vi "BSCAN_DEMO00_init_xc7z020_clg400.vi"() -> ()   [LabVIEW 2017]
doc: "Copyright © 2024 SalDigi Oy, all rights reserved."
uses:
  Saldigi_protocol_library.lvlibp/HAL/HAL_version_typedef.ctl
  Saldigi_protocol_library.lvlibp/BSCAN_bitstream/private/BSCAN_INSTRUCTION_OPCODE_typedef.ctl
  Saldigi_protocol_library.lvlibp/BSCAN_bitstream/BSCAN_typedef.ctl
  Saldigi_protocol_library.lvlibp/BSCAN_bitstream/BSCAN_state_typedef.ctl
  Saldigi_protocol_library.lvlibp/BSCAN_bitstream/simultaneous/BSCAN_extest_dataToInject.ctl
  Saldigi_protocol_library.lvlibp
panel:
  in  "TAPs OPCODE array (use only BYPASS or EXTEST here)":T1[](array[typedef])=[enum."BYPASS", enum."EXTEST"]
  in  "HAL Version":T2=enum."FTn232H"
  in  "Init output rate":dbl=1000000.0 format="%^#_6g"
  in  "Start V2 Server":bool
  out "shift-IR OK":bool
  out "ID registers from BSDL out (string)":string[](array[string])
  out "ID registers out (U32)":u32[](array[numeric]) format="%032b"
  in  "CHAINn name in":string(combo)="chain0"
  in  "Parameter string":string(combo)="FTERYEPB"
  in  "TDO-in channel name":string(combo)="D3"
  in  "TCK channel name":string(combo)="D0"
  in  "TDI channel name":string(combo)="D1"
  in  "TMS channel name":string(combo)="D6"
  in  "output rate":dbl=10000000.0 format="%^#_6g"
  in  "BSDL files in":path[](array[path])=[path "C:/bitstream/zynq7000_arm_dap.bsd", path "C:/bitstream/xc7z020_clg400.bsd"]
  out "error out":errorcluster
  in  "error in":errorcluster
  out "ALL TAPs IDCODE OK":bool
  # "First TAP in CHAINn is on array index[0]."
  # "The combo boxes below include examples for DAQmx and FTn232H. Edit these to suit your\nsystem."
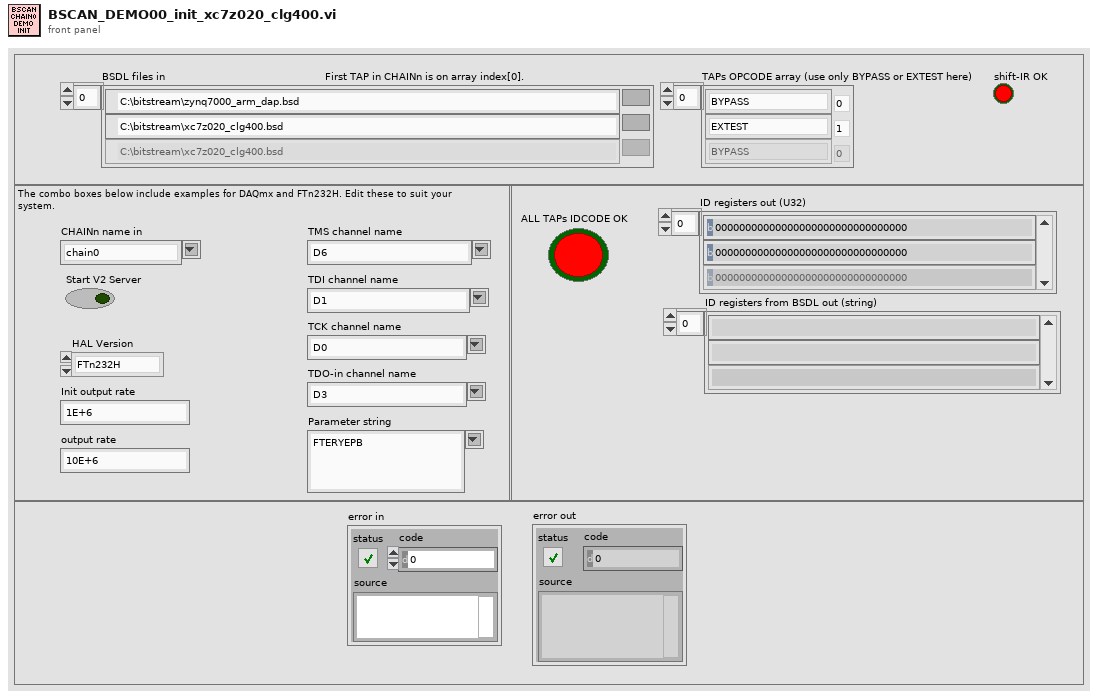
[diagram p1: front panel]
types:
  T1 = typedef "Saldigi_protocol_library.lvlibp/BSCAN_INSTRUCTION_OPCODE_typedef.ctl" = enum16{"BYPASS", "EXTEST", "PRELOAD", "SAMPLE", "CLAMP", "HIGHZ", "INTEST", "RUNBIST", "USERCODE", "IDCODE"}
  T2 = typedef "Saldigi_protocol_library.lvlibp/HAL_version_typedef.ctl" = enum16{"DAQmx V1", "DAQmx V2", "FTn232H", "BSCAN V1", "DAQmx V1.1", "DAQmx V2.1", "J-LINK BSCAN", "BSCAN V2"}
  T3 = typedef "Saldigi_protocol_library.lvlibp/BSCAN_typedef.ctl" = cluster{"TMS":bool[], "TDI":bool[], "TCK":bool[], "TDO-in":bool[], "clocked bits":i32, "output rate":dbl, "TMS channel name":string, "TDI channel name":string, "TCK channel name":string, "TDO-in channel name":string, "Parameter string":string, "String array":string[], "State":T4, "CHAINn":string, "Version":T2, "V2 Server queue":refnum<queue>, "V2 max client \ndata array length":i32}
  T4 = typedef "Saldigi_protocol_library.lvlibp/BSCAN_state_typedef.ctl" = enum16{"Test-Logic-Reset", "Run-Test/Idle", "Select DR-Scan", "Capture-DR", "Shift-DR", "Exit1-DR", "Pause-DR", "Exit2-DR", "Update-DR", "Select-IR-Scan", "Capture-IR", "Shift-IR", "Exit1-IR", "Pause-IR", "Exit2-IR", "Update-IR"}
  T5 = cluster{"CHAINn/TARGETn/PORTn in":string[], "port states in":bool[], "port driver states in":enum16{"Enable driver", "Disable driver", "Read"}[]}
  T6 = enum16{"Enable driver", "Disable driver", "Read"}[]
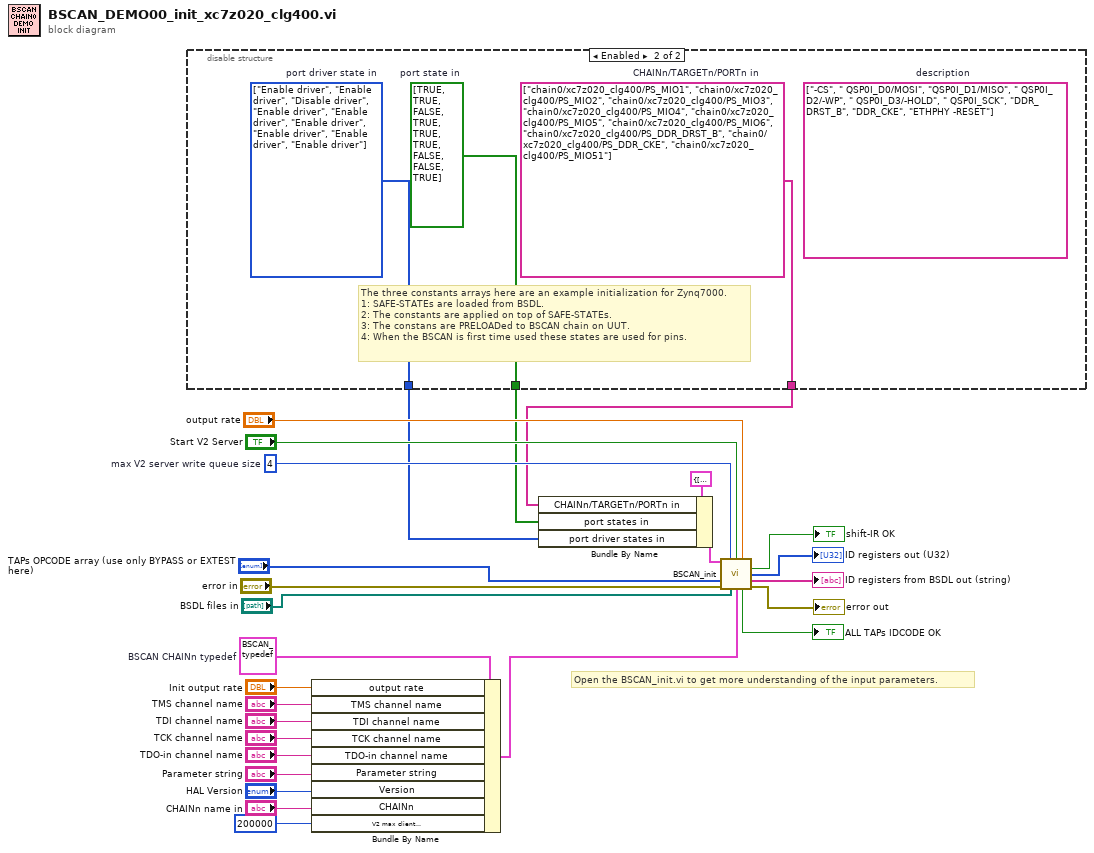
[diagram p0: block diagram]
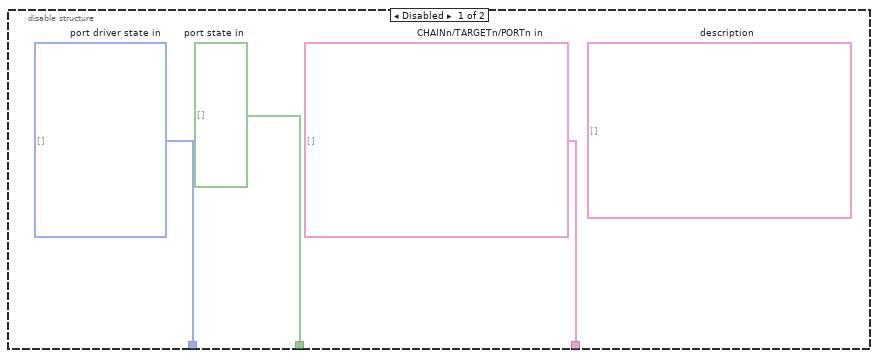
[diagram p2: hidden frame]
diagram:
  w2 = T3 {"TMS"=[], "TDI"=[], "TCK"=[], "TDO-in"=[], "clocked bits"=0, "output rate"=0.0, "TMS channel name"="", "TDI channel name"="", "TCK channel name"="", "TDO-in channel name"="", "Parameter string"="", "String array"=[], "State"=enum."Test-Logic-Reset", "CHAINn"="chain0", "Version"=enum."FTn232H", "V2 Server queue"=refnum, "V2 max client \ndata array length"=0}  # BSCAN CHAINn typedef
  w21 = 4  # max V2 server write queue size
  # "Open the BSCAN_init.vi to get more understanding of the input parameters."
  n1 = disable-structure shown="Enabled" {
    disable-tunnel: [w30 w33] -> w9
    disable-tunnel: [w29 w32] -> w8
    disable-tunnel: [w28 w31] -> w7
    frame Disabled {
      (unwired) string[] []  # description
      w29 = bool[] []  # port state in
      w28 = T6 [] items=["Enable driver", "Disable driver", "Read"]  # port driver state in
      w30 = string[] []  # CHAINn/TARGETn/PORTn in
    }
    frame Enabled {
      (unwired) string[] ["-CS", " QSP0I_D0/MOSI", "QSP0I_D1/MISO", " QSP0I_D2/-WP", " QSP0I_D3/-HOLD", " QSP0I_SCK", "DDR_DRST_B", "DDR_CKE", "ETHPHY -RESET"]  # description
      w32 = bool[] [TRUE, TRUE, FALSE, TRUE, TRUE, TRUE, FALSE, FALSE, TRUE]  # port state in
      w31 = T6 [enum."Enable driver", enum."Enable driver", enum."Disable driver", enum."Enable driver", enum."Enable driver", enum."Enable driver", enum."Enable driver", enum."Enable driver", enum."Enable driver"] items=["Enable driver", "Disable driver", "Read"]  # port driver state in
      w33 = string[] ["chain0/xc7z020_clg400/PS_MIO1", "chain0/xc7z020_clg400/PS_MIO2", "chain0/xc7z020_clg400/PS_MIO3", "chain0/xc7z020_clg400/PS_MIO4", "chain0/xc7z020_clg400/PS_MIO5", "chain0/xc7z020_clg400/PS_MIO6", "chain0/xc7z020_clg400/PS_DDR_DRST_B", "chain0/xc7z020_clg400/PS_DDR_CKE", "chain0/xc7z020_clg400/PS_MIO51"]  # CHAINn/TARGETn/PORTn in
      # "The three constants arrays here are an example initialization for Zynq7000.\n1: SAFE-STATEs are loaded from BSDL.\n2: The constants are applied on top of SAFE-STATEs.\n3: The constans are PRELOADed to BSCAN chain on UUT.\n4: When the BSCAN is first time used these states are used for pins."
    }
  }
  n2 = Bundle By Name(cluster=w2, "output rate"="Init output rate", "TMS channel name"="TMS channel name", "TDI channel name"="TDI channel name", "TCK channel name"="TCK channel name", "TDO-in channel name"="TDO-in channel name", "Parameter string"="Parameter string", "Version"="HAL Version", "CHAINn"="CHAINn name in", "V2 max client \ndata array length"=200000 ("V2 max client \ndata array length")) -> (w1:T3)
  n3 = Bundle By Name(cluster=T5 {"CHAINn/TARGETn/PORTn in"=[], "port states in"=[], "port driver states in"=[]} ("UserConfig on top of SAFE-STATEs"), "CHAINn/TARGETn/PORTn in"=w9, "port states in"=w8, "port driver states in"=w7) -> (w5:T5)
  n4 = call "BSCAN_init.vi"("UserConfig on top of SAFE-STATEs"=w5, "max V2 server write queue size"=w21, "Start V2 Server"="Start V2 Server", "output rate"="output rate", "TAPs OPCODE array\n(use only BYPASS or EXTEST here)"="TAPs OPCODE array (use only BYPASS or EXTEST here)", "error in (no error)"="error in", "BSDL files in"="BSDL files in", "BSCAN CHAINn typedef"=w1) -> ("shift-IR OK"=→"shift-IR OK":bool, "ID registers out (U32)"=→"ID registers out (U32)":u32[], "ID registers from BSDL out (string)"=→"ID registers from BSDL out (string)":string[], "ALL TAPs IDCODE OK"=→"ALL TAPs IDCODE OK":bool, "error out"=→"error out":errorcluster)  [unwired: 3 in]
